vi "Simulation.vi"(0 "FPGA API Mock in":refnum<class "FPGA API Mock.lvclass">, 11 "error in (no error)":errorcluster) -> (4 "FPGA API Mock out":refnum<class "FPGA API Mock.lvclass">, 15 "error out":errorcluster)   [LabVIEW 2019, in "FPGA API Mock.lvclass"]
uses:
  FPGA API Mock.lvclass
  FPGA API Mock.lvclass/FPGA API Mock.ctl
  <vilib>/ptbypt/NI_PtbyPt.lvlib
panel:
  in  "index":i32
  in  "RESET DO":bool
  in  "SET DO":bool
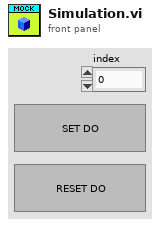
[diagram p1: front panel]
types:
  T1 = typedef "FPGA API Mock.lvclass/Data.ctl" = cluster{"DO":bool[], "DI":bool[], "AI":dbl[], "AO":dbl[]}
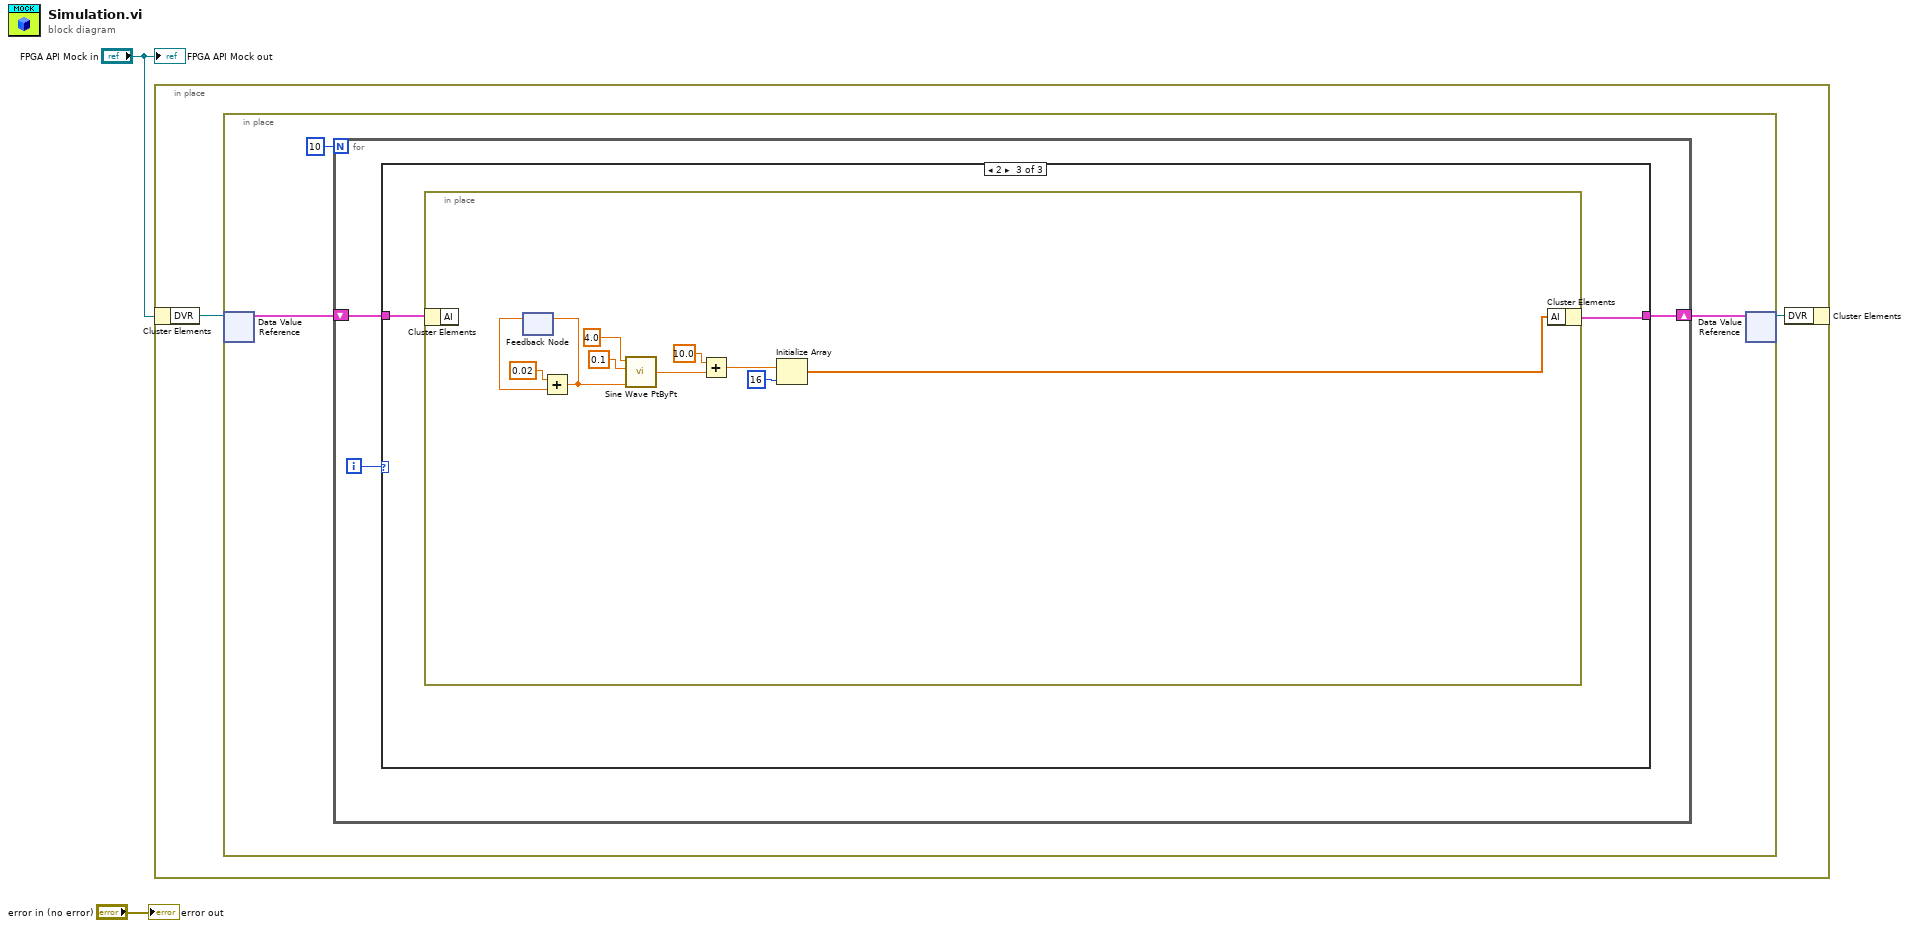
[diagram p0: block diagram]
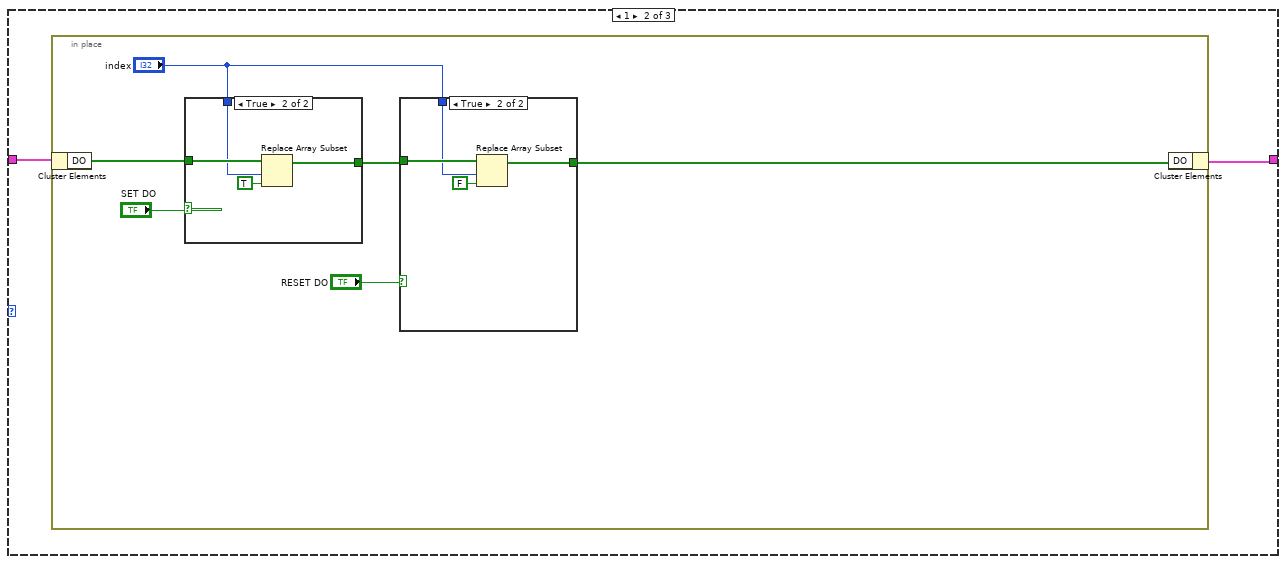
[diagram p3: hidden frame]
diagram:
  n1 = in-place {
    n2 = in-place-cluster #1("FPGA API Mock in") -> ("DVR"=w4:refnum<data-value>)
    n3 = in-place {
      n4 = in-place-dvr #2(w4) -> (w7:T1)  [unwired: 1 out]
      n5 = for {
        N: 10 -> [_]
        shift-right: [w9] -> w6
        shift-left: w7 -> [w10]
        i -> [w8]
        n6 = case shown="2" w8 {
          tunnel: w10 -> [w11 w13 w31]
          tunnel: [w11 w12 w30] -> w9
          frame Default {
          }
          frame 1 {
            n7 = in-place {
              n8 = in-place-cluster #3(w13) -> ("DO"=w19:bool[])
              n9 = case shown="True" "SET DO" {
                tunnel: w19 -> [w25 w29]
                tunnel: "index" -> [_ w28]
                tunnel: [w25 w26] -> w17
                frame False {
                }
                frame True {
                  n10 = Replace Array Subset(array=w29, new element=TRUE ("new element/subarray"), index=w28) -> (w26:bool[])
                }
              }
              n11 = case shown="True" "RESET DO" {
                tunnel: w17 -> [w20 w24]
                tunnel: "index" -> [_ w23]
                tunnel: [w20 w21] -> w15
                frame False {
                }
                frame True {
                  n12 = Replace Array Subset(array=w24, new element=FALSE ("new element/subarray"), index=w23) -> (w21:bool[])
                }
              }
              n13 = in-place-cluster #3("DO"=w15) -> (w12:T1)
            }
          }
          frame 2 {
            n14 = in-place {
              n15 = in-place-cluster #4(w31) -> ()  [unwired: 1 out]
              n16 = feedback #5() -> (w37:dbl)  [unwired: 1 in]
              n17 = Add(x=0.02, y=w37) -> (x+y=w35:dbl)
              n18 = feedback-in #5(w35) -> ()
              n19 = call <vilib>:"Sine Wave PtByPt.vi"("time"=w35, "frequency"=0.1, "amplitude"=4.0) -> ("sine wave"=w39:dbl)  [unwired: 1 in]
              n20 = Add(x=10.0, y=w39) -> (x+y=w34:dbl)
              n21 = Initialize Array(w34, 16 ("dimension size")) -> (w32:dbl[])
              n22 = in-place-cluster #4("AI"=w32) -> (w30:T1)
            }
          }
        }
      }
      n23 = in-place-dvr #2(w6) -> (w3:refnum<data-value>)  [unwired: 1 out]
    }
    n24 = in-place-cluster #1("DVR"=w3) -> ()  [unwired: 1 out]
  }
  "error out" <- "error in (no error)"
  "FPGA API Mock out" <- "FPGA API Mock in"
